vi "GUI.vi"() -> ()   [LabVIEW 2019]
panel:
  in  "Stop":bool
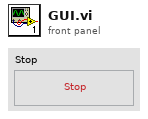
[diagram p1: front panel]
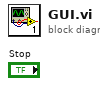
[diagram p0: block diagram]
diagram:
